vi "DVR Performance Test.vi"() -> ()   [LabVIEW 2021]
panel:
  out "x-y":dbl format="%#_6p"
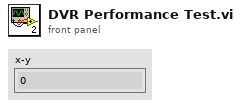
[diagram p1: front panel]
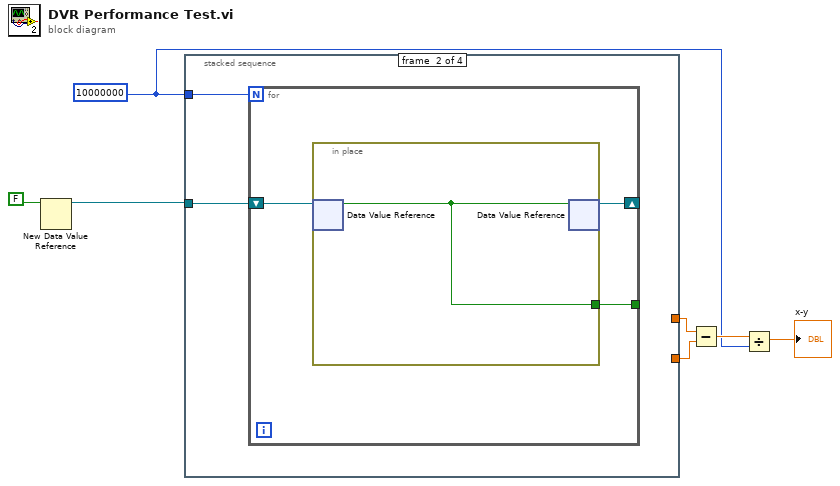
[diagram p0: block diagram]
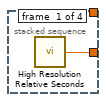
[diagram p2: hidden frame]
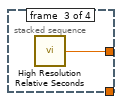
[diagram p3: hidden frame]
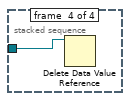
[diagram p4: hidden frame]
diagram:
  w3 = 10000000
  n1 = New Data Value Reference(data value=FALSE) -> (data value reference=w2:refnum<data-value>)  [unwired: 1 in, 1 out]
  n2 = stacked-sequence {
    tunnel: w2 -> [_ w10 _ w16]
    tunnel: [w8 _ _ _] -> w7
    tunnel: [_ _ w15 _] -> w6
    tunnel: w3 -> [_ w9 _ _]
    frame #0 {
      n3 = call <vilib>:"High Resolution Relative Seconds.vi"() -> ("relative seconds"=w8:dbl)
    }
    frame #1 {
      n4 = for {
        N: w9 -> [_]
        tunnel: [w12] -> _
        shift-right: [w11] -> _
        shift-left: w10 -> [w13]
        n5 = in-place {
          in-place-border: [w14] -> w12
          n6 = in-place-dvr #1(w13) -> (w14:bool)  [unwired: 1 out]
          n7 = in-place-dvr #1(w14) -> (w11:refnum<data-value>)  [unwired: 1 out]
        }
      }
    }
    frame #2 {
      n8 = call <vilib>:"High Resolution Relative Seconds.vi"() -> ("relative seconds"=w15:dbl)
    }
    frame #3 {
      n9 = Delete Data Value Reference(data value reference=w16) -> ()  [unwired: 1 in, 2 out]
    }
  }
  n10 = Subtract(x=w6, y=w7) -> (x-y=w5:dbl)
  n11 = Divide(x=w5, y=w3) -> (x/y=→"x-y":dbl)
